vi "FPGA_EncoderOpen.vi"   [LabVIEW 2017]
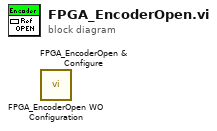
[diagram p0: block diagram]
diagram:
  n1 = call <vilib>:"FPGA_EncoderOpen WO Configuration.vi"() -> ()  [unwired: 10 in, 2 out]
  n2 = call <vilib>:"FPGA_EncoderOpen & Configure.vi"() -> ()  [unwired: 10 in, 2 out]
